vi "TEST - Clear All Errors.vi"(8 "error in (no error)":errorcluster) -> (0 "error out":errorcluster, 2 "pass":bool)   [LabVIEW 2020]
uses:
  source/library/openg_error.lvlib
  <vilib>/addons/_JKI Toolkits/Caraya/classes/Assert/Assert.lvclass
  <vilib>/addons/_JKI Toolkits/Caraya/classes/Test/Test.lvclass
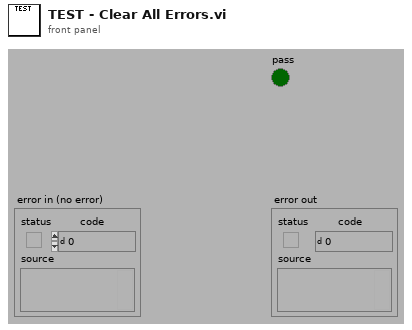
[diagram p1: front panel]
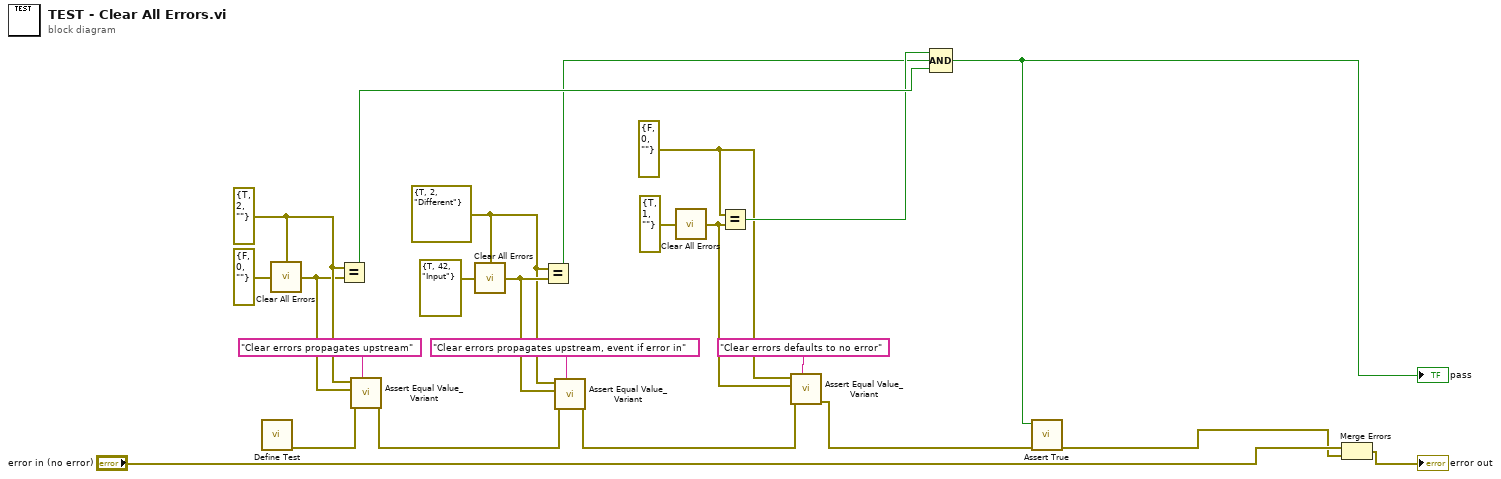
[diagram p0: block diagram]
diagram:
  w6 = errorcluster {"status"=TRUE, "code"=2, "source"="Different"} ("Upsteam Error (optional)")
  w13 = errorcluster {"status"=FALSE, "code"=0, "source"=""} ("Error In")
  w16 = errorcluster {"status"=TRUE, "code"=2, "source"=""} ("Upsteam Error (optional)")
  n1 = call <vilib>:"Define Test.vi"() -> ("error out"=w14:errorcluster)  [unwired: 11 in]
  n2 = call "Clear All Errors.vi"("Upsteam Error (optional)"=w16, "Error In"=errorcluster {"status"=FALSE, "code"=0, "source"=""}) -> ("Error Out"=w15:errorcluster)  [unwired: 2 in]
  n3 = Equal?(x=w16, y=w15) -> (x = y?=w20:bool)
  n4 = call <vilib>:"Assert Equal Value_Variant.vi"("Label"="Clear errors propagates upstream", "error in (no error)"=w14, "Y"=w15, "X"=w16) -> ("error out"=w3:errorcluster)  [unwired: 7 in]
  n5 = call "Clear All Errors.vi"("Upsteam Error (optional)"=w6, "Error In"=errorcluster {"status"=TRUE, "code"=42, "source"="Input"}) -> ("Error Out"=w7:errorcluster)  [unwired: 2 in]
  n6 = Equal?(x=w6, y=w7) -> (x = y?=w4:bool)
  n7 = call <vilib>:"Assert Equal Value_Variant.vi"("Label"="Clear errors propagates upstream, event if error in", "error in (no error)"=w3, "Y"=w7, "X"=w6) -> ("error out"=w2:errorcluster)  [unwired: 7 in]
  n8 = call "Clear All Errors.vi"("Error In"=errorcluster {"status"=TRUE, "code"=1, "source"=""}) -> ("Error Out"=w12:errorcluster)  [unwired: 3 in]
  n9 = Equal?(x=w13, y=w12) -> (x = y?=w18:bool)
  n10 = call <vilib>:"Assert Equal Value_Variant.vi"("Label"="Clear errors defaults to no error", "error in (no error)"=w2, "Y"=w12, "X"=w13) -> ("error out"=w11:errorcluster)  [unwired: 7 in]
  n11 = Compound Arithmetic op=AND(w18, w4, w20) -> (w17:bool)
  "pass" <- w17
  n12 = call <vilib>:"Assert True.vi"("error in (no error)"=w11, "True?"=w17) -> ("error out"=w1:errorcluster)  [unwired: 9 in]
  n13 = Merge Errors("error in (no error)", w1) -> (→"error out":errorcluster)
